vi "Load_STS_param_options.vi"(9 "load":u16(ring) items=["numerical_-1V->2V", "numerical_-20mV->20mV", "numerical_-2V->2.2V", "lockin_-20mV->20mV", "lockin_-25mV->25mV", "test", "lockin_highRes_20mV_-20mV", "lockin_slow", "Lock_in_DCA_1.5V->-50mV", "Long_MgPc_lockin_-1->1V", "MgPc_long_lockin", "lockin_slow_-1_2", "MgPc_long_lockin2", "Quick_Lockin"]) -> (3 "STSTypes []":string[](array[string]))   [LabVIEW 2014]
panel:
  out "loaded":i32
  out "data":T1(array[cluster])
  # "make sure\nLockin is activated\nin Advanced Settings"
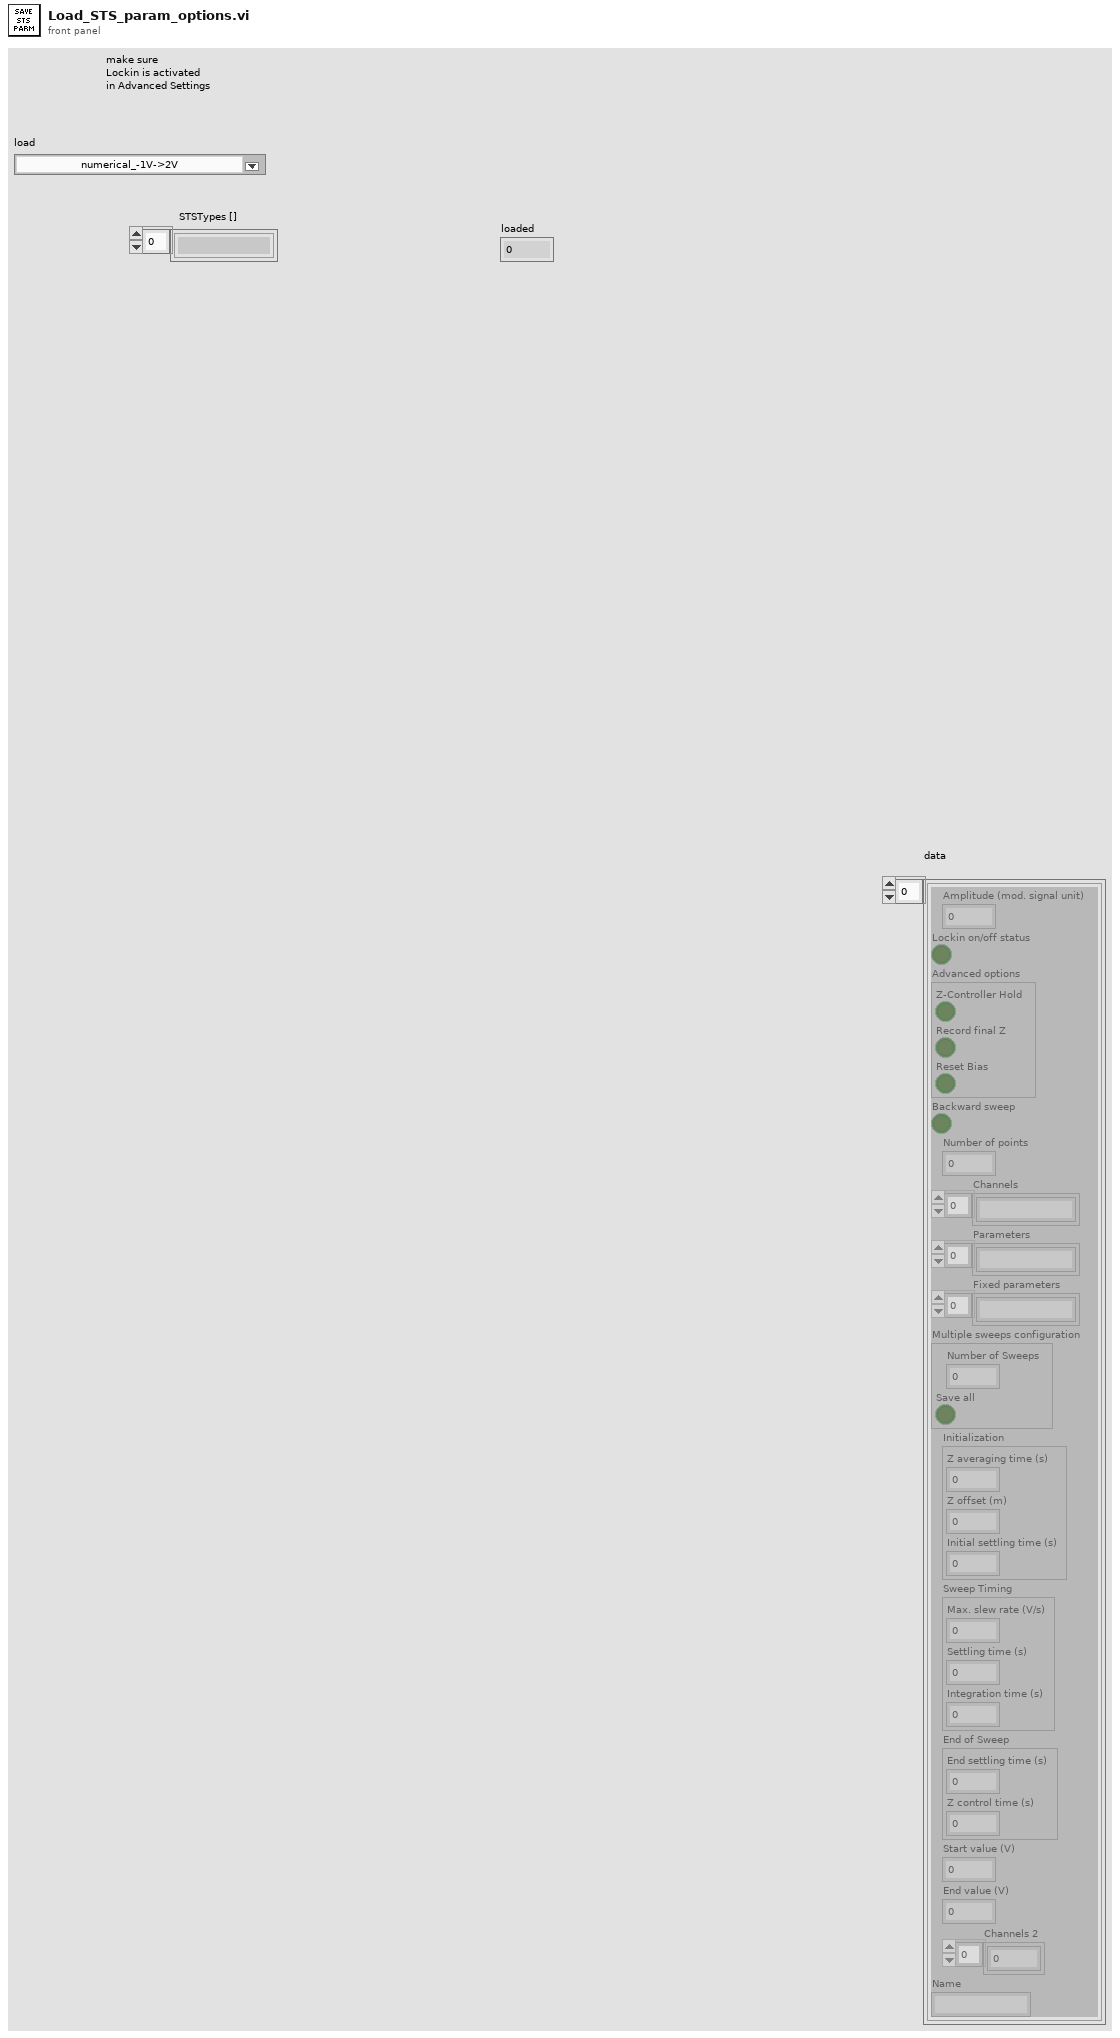
[diagram p1: front panel]
types:
  T1 = cluster{"Amplitude (mod. signal unit)":sgl, "Lockin on/off status":bool, "Advanced options":cluster{"Z-Controller Hold":bool, "Record final Z":bool, "Reset Bias":bool}, "Backward sweep":bool, "Number of points":i32, "Channels":string[], "Parameters":string[], "Fixed parameters":string[], "Multiple sweeps configuration":cluster{"Number of Sweeps":i32, "Save all":bool}, "Initialization":cluster{"Z averaging time (s)":sgl, "Z offset (m)":sgl, "Initial settling time (s)":sgl}, "Sweep Timing":cluster{"Max. slew rate (V/s)":sgl, "Settling time (s)":sgl, "Integration time (s)":sgl}, "End of Sweep":cluster{"End settling time (s)":sgl, "Z control time (s)":sgl}, "Start value (V)":sgl, "End value (V)":sgl, "Channels 2":i32[], "Name":string}[]
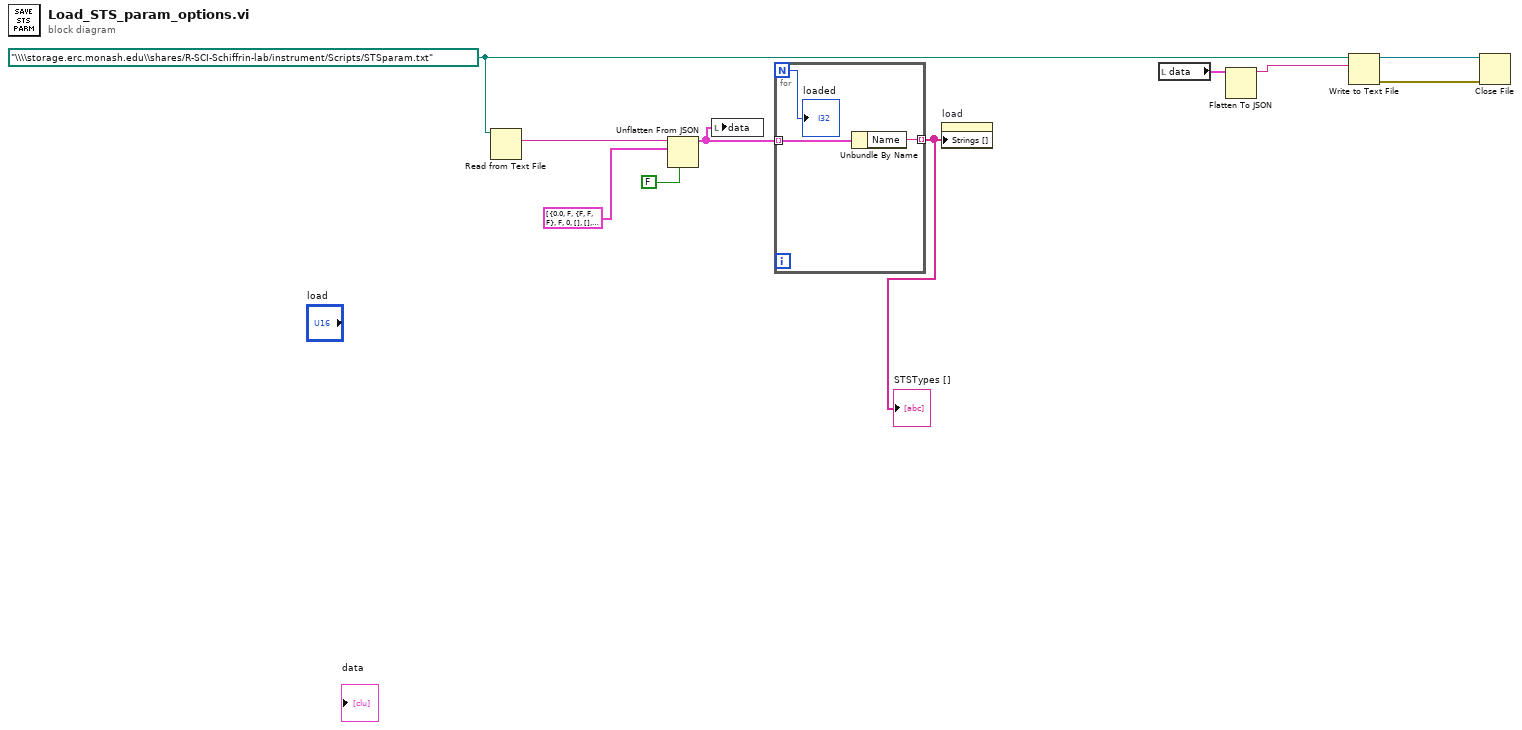
[diagram p0: block diagram]
diagram:
  w10 = path "\\\\storage.erc.monash.edu\\shares/R-SCI-Schiffrin-lab/instrument/Scripts/STSparam.txt" ("file (use dialog)")
  n1 = Read from Text File(file (use dialog)=w10) -> (text=w9:string)  [unwired: 3 in, 3 out]
  n2 = Unflatten From JSON(JSON string=w9, type and defaults=T1 [{"Amplitude (mod. signal unit)"=0.0, "Lockin on/off status"=FALSE, "Advanced options"={"Z-Controller Hold"=FALSE, "Record final Z"=FALSE, "Reset Bias"=FALSE}, "Backward sweep"=FALSE, "Number of points"=0, "Channels"=[], "Parameters"=[], "Fixed parameters"=[], "Multiple sweeps configuration"={"Number of Sweeps"=0, "Save all"=FALSE}, "Initialization"={"Z averaging time (s)"=0.0, "Z offset (m)"=0.0, "Initial settling time (s)"=0.0}, "Sweep Timing"={"Max. slew rate (V/s)"=0.0, "Settling time (s)"=0.0, "Integration time (s)"=0.0}, "End of Sweep"={"End settling time (s)"=0.0, "Z control time (s)"=0.0}, "Start value (V)"=0.0, "End value (V)"=0.0, "Channels 2"=[], "Name"=""}, {"Amplitude (mod. signal unit)"=0.0015, "Lockin on/off status"=FALSE, "Advanced options"={"Z-Controller Hold"=TRUE, "Record final Z"=FALSE, "Reset Bias"=TRUE}, "Backward sweep"=TRUE, "Number of points"=128, "Channels"=["Current (A)", "LI Demod 1 X (A)", "LI Demod 1 Y (A)", "LI Demod 2 X (A)", "LI Demod 2 Y (A)"], "Parameters"=["X (m)", "Y (m)", "Z (m)", "Z offset (m)", "Settling time (s)", "Integration time (s)", "Z-Ctrl hold", "Final Z (m)"], "Fixed parameters"=["Sweep Start", "Sweep End"], "Multiple sweeps configuration"={"Number of Sweeps"=100, "Save all"=FALSE}, "Initialization"={"Z averaging time (s)"=0.001, "Z offset (m)"=0.0, "Initial settling time (s)"=5e-05}, "Sweep Timing"={"Max. slew rate (V/s)"=inf, "Settling time (s)"=0.001, "Integration time (s)"=0.0005}, "End of Sweep"={"End settling time (s)"=5e-05, "Z control time (s)"=0.0}, "Start value (V)"=-0.02, "End value (V)"=0.02, "Channels 2"=[0, 20, 21, 22, 23], "Name"="Numerical_-20mV->20mV"}] ("data"), default null elements? (F)=FALSE) -> (value=w6:T1)  [unwired: 4 in, 1 out]
  n3 = local write "data"(w6) -> ()
  n4 = for {
    N -> [w11]
    tunnel: w6 -> [w13] mode=indexing
    tunnel: [w12] -> w5 mode=indexing
    n5 = Unbundle By Name(w13) -> ("Name"=w12:string)
    "loaded" <- w11
  }
  "STSTypes []" <- w5
  n6 = property on="load" class="Ring (strict)"("Strings []"=w5) -> ()  [unwired: 2 in, 2 out]
  n7 = local read "data"() -> (w1:T1)
  n8 = Flatten To JSON(anything=w1) -> (JSON string=w4:string)  [unwired: 2 in, 1 out]
  n9 = Write to Text File(file (use dialog)=w10, text=w4) -> (refnum out=w2:refnum<file>, error out=w3:errorcluster)  [unwired: 2 in, 1 out]
  n10 = Close File(refnum=w2, error in=w3) -> ()  [unwired: 2 out]
